vi "Motor_Read_Velocity.vi"(0 "VISA resource IN":refnum<visa-resource-name>, 5 "Motor Bus Address to  Read":u8, 11 "error in (no error)":errorcluster) -> (4 "VISA resource OUT":refnum<visa-resource-name>, 6 "Native Units (VT)":i32, 8 "Revolutions Per Second (RPS)":dbl, 10 "Revolutions Per Minute (RPM)":dbl, 15 "error out":errorcluster)   [LabVIEW 2017]
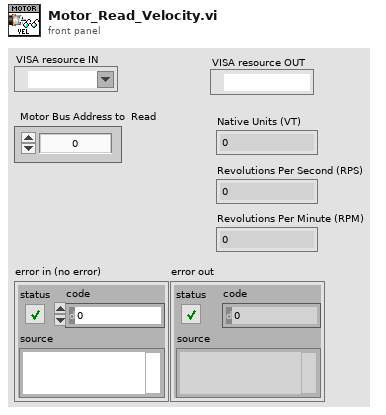
[diagram p1: front panel]
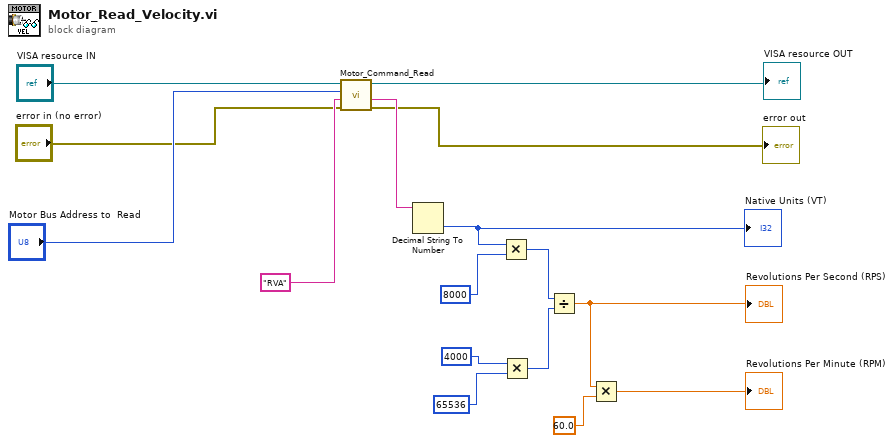
[diagram p0: block diagram]
diagram:
  n1 = call "Motor_Command_Read.vi"("VISA resource IN"="VISA resource IN", "Motor Number"="Motor Bus Address to  Read", "Read Command to Motor"="RVA", "Error In"="error in (no error)") -> ("VISA resource OUT"=→"VISA resource OUT":refnum<visa-resource-name>, "Response From Motor"=w9:string, "Error Out"=→"error out":errorcluster)  [unwired: 2 in, 1 out]
  n2 = Decimal String To Number(string=w9) -> (number=w3:i32)  [unwired: 2 in, 1 out]
  "Native Units (VT)" <- w3
  n3 = Multiply(x=w3, y=8000) -> (x*y=w13:i32)
  n4 = Multiply(x=4000, y=65536) -> (x*y=w14:i32)
  n5 = Divide(x=w13, y=w14) -> (x/y=w8:dbl)
  "Revolutions Per Second (RPS)" <- w8
  n6 = Multiply(x=w8, y=60.0) -> (x*y=→"Revolutions Per Minute (RPM)":dbl)
